vi "Parse State from Frame Name.vi"(7 "Category (Optional)":string, 11 "Frame or State Name":string) -> (0 "Has Category?":bool, 1 "is a Category Frame?":bool, 2 "State Name":string, 3 "Category Name":string, 4 "\"Category: State\" String":string)   [LabVIEW 2013, in "JKI State Machine API.lvlib" / "JKI SM.lvclass"]
uses:
  JKI SM.lvclass
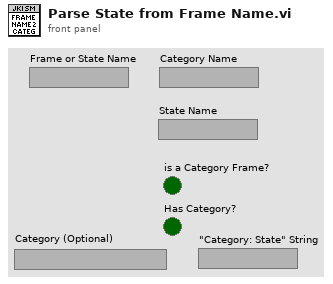
[diagram p1: front panel]
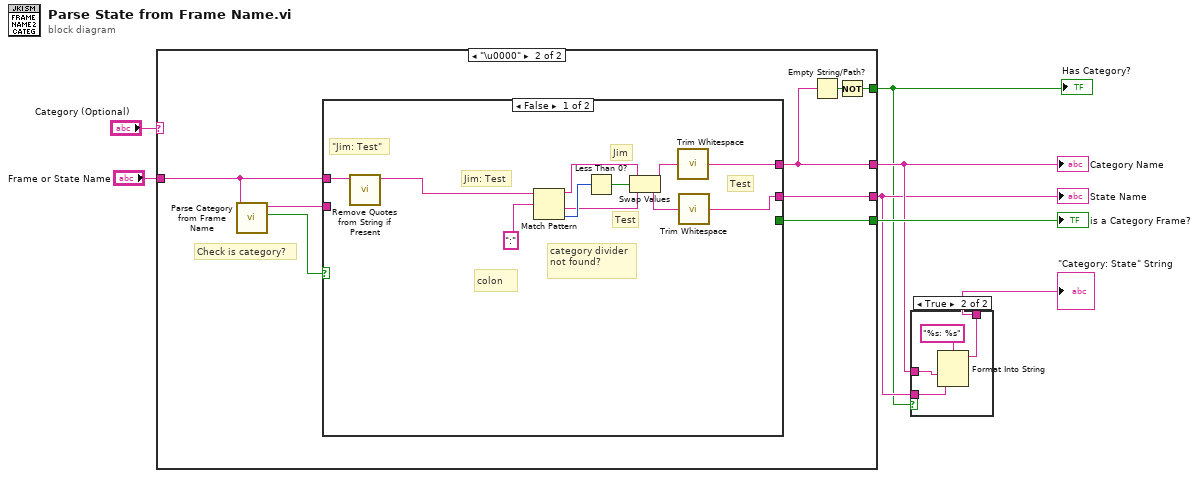
[diagram p0: block diagram]
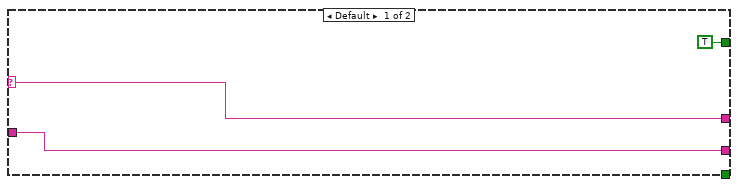
[diagram p2: hidden frame]
diagram:
  n1 = case shown="\"\"" "Category (Optional)" {
    selector: "Category (Optional)" -> [w10 _]
    tunnel: "Frame or State Name" -> [w9 w17]
    tunnel: [TRUE w15] -> w1
    tunnel: [_ w13] -> w6
    tunnel: [w10 w12] -> w5
    tunnel: [w9 w11] -> w4
    frame Default {
    }
    frame "\u0000" {
      # "Check is category?"
      n2 = call "Parse Category from Frame Name.vi"("Frame Name"=w17) -> ("is a Category?"=w18:bool, "Category Name"=w14:string)  [unwired: 9 in]
      n3 = case shown="False" w18 {
        selector: w18 -> [_ w31]
        tunnel: [_ w31] -> w13
        tunnel: [w25 w30] -> w12
        tunnel: w14 -> [_ w30]
        tunnel: w17 -> [w28 _]
        tunnel: [w26 _] -> w11
        frame False {
          # "category divider not found?"
          # "Test"
          # "Test"
          # "Jim"
          # "Jim: Test"
          # "\"Jim: Test\""
          # "colon"
          n4 = call "Remove Quotes from String if Present.vi"("String"=w28) -> ("String with Quotes Removed"=w27:string)  [unwired: 10 in]
          n5 = Match Pattern(string=w27, regular expression=":") -> (before substring=w22:string, after substring=w20:string, offset past match=w24:i32)  [unwired: 1 in, 1 out]
          n6 = Less Than 0?(x=w24) -> (x < 0?=w23:bool)
          n7 = Swap Values(12:w22, 13:w23, 14:w20) -> (1:w21:string, 3:w19:string)
          n8 = call <vilib>:"Trim Whitespace.vi"("string"=w21) -> ("trimmed string"=w25:string)  [unwired: 1 in]
          n9 = call <vilib>:"Trim Whitespace.vi"("string"=w19) -> ("trimmed string"=w26:string)  [unwired: 1 in]
        }
        frame True {
        }
      }
      n10 = Empty String/Path?(string/path=w12) -> (empty?=w16:bool)
      n11 = Not(x=w16) -> (.not. x?=w15:bool)
    }
  }
  "is a Category Frame?" <- w6
  "Category Name" <- w5
  "State Name" <- w4
  "Has Category?" <- w1
  n12 = case shown="True" w1 {
    tunnel: w4 -> [w32 w36]
    tunnel: w5 -> [_ w35]
    tunnel: [w32 w33] -> w3
    frame False {
    }
    frame True {
      n13 = Format Into String(format string="%s: %s", w35, w36) -> (resulting string=w33:string)  [unwired: 2 in, 1 out]
    }
  }
  "\"Category: State\" String" <- w3
